vi "KGN Set Pump Concentrations.vi"(6 "Pump Concentrations-Cluster":T1(array[cluster]), 7 "scaling":dbl=1000000.0, 8 "Fehler (Eingang, kein Fehler)":errorcluster, 9 "Info Cluster":T2, 10 "VISA-Referenz (Eingang)":refnum<visa-resource-name>, 11 "device (Eingang)":u32) -> (0 "Fehler (Ausgang)":errorcluster, 1 "Info Cluster out":T2, 2 "VISA-Referenz (Ausgang)":refnum<visa-resource-name>, 3 "dup device (Ausgang)":u32, 4 "Kommandos gesendet":string)   [LabVIEW 2020, in "Linearisierung v2.lvlib" / "Gasteiler.lvlib" / "HovaCAL_Interface.lvlib" / "KGN.lvlib" / "KGN GUI Set.lvlib"]
uses:
  KGN GUI Set.lvlib
  Controls/Info Cluster.ctl
  set/set.lvlib
  Controls/Controls.lvlib
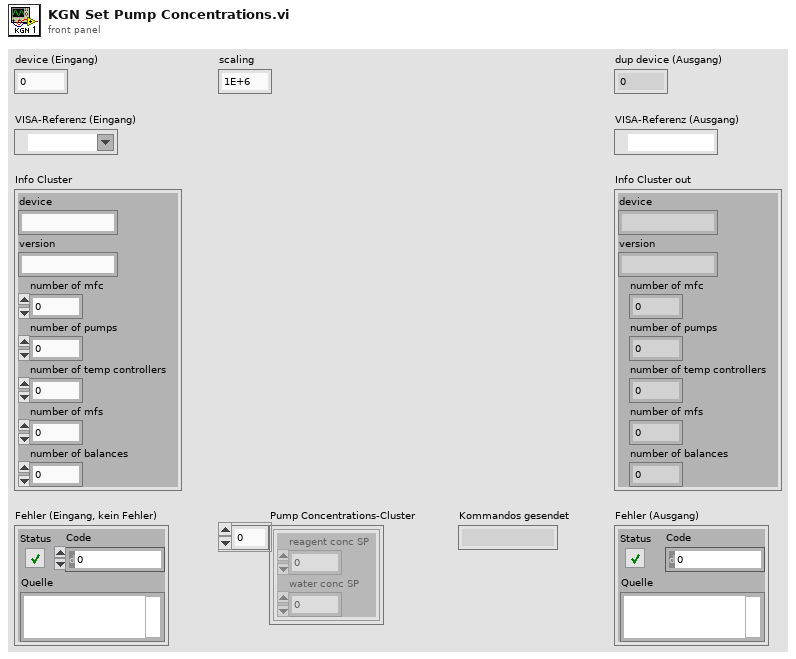
[diagram p1: front panel]
types:
  T1 = cluster{"reagent conc SP":dbl, "water conc SP":dbl}[]
  T2 = typedef "Linearisierung v2.lvlib/Gasteiler.lvlib/HovaCAL_Interface.lvlib/Controls.lvlib/Info Cluster.ctl" = cluster{"device":string, "version":string, "number of mfc":i32, "number of pumps":i32, "number of temp controllers":i32, "number of mfs":i32, "number of balances":i32}
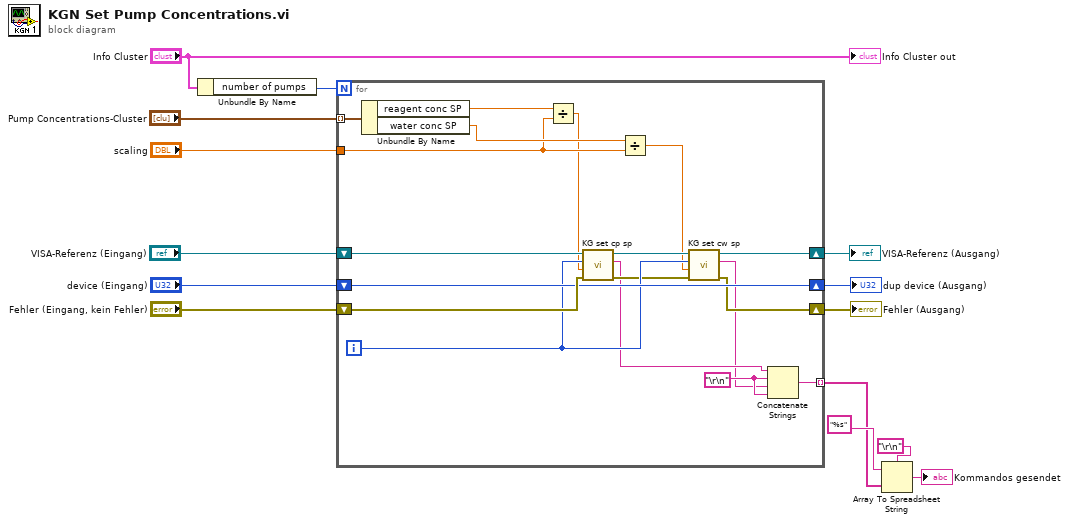
[diagram p0: block diagram]
diagram:
  n1 = Unbundle By Name("Info Cluster") -> ("number of pumps"=w9:i32)
  n2 = for {
    N: w9 -> [_]
    shift-right: [w31] -> w12
    shift-left: "device (Eingang)" -> [w31]
    shift-right: [w30] -> w11
    shift-left: "Fehler (Eingang, kein Fehler)" -> [w32]
    tunnel: "scaling" -> [w20]
    tunnel: "Pump Concentrations-Cluster" -> [w28] mode=indexing
    shift-right: [w25] -> w5
    shift-left: "VISA-Referenz (Eingang)" -> [w26]
    tunnel: [w15] -> w2 mode=indexing
    i -> [w29]
    w18 = "\r\n"
    n3 = Unbundle By Name(w28) -> ("reagent conc SP"=w21:dbl, "water conc SP"=w27:dbl)
    n4 = Divide(x=w21, y=w20) -> (x/y=w19:dbl)
    n5 = call "KG set cp sp.vi"("Fehler (Eingang, kein Fehler)"=w32, "Concentration"=w19, "pump"=w29, "VISA-Ressourcenname"=w26) -> ("Fehler (Ausgang)"=w23:errorcluster, "Kommando gesendet"=w17:string, "VISA-Ressourcenname (Ausgang)"=w24:refnum<visa-resource-name>)  [unwired: 5 in]
    n6 = Divide(x=w27, y=w20) -> (x/y=w22:dbl)
    n7 = call "KG set cw sp.vi"("Fehler (Eingang, kein Fehler)"=w23, "Concentration"=w22, "pump"=w29, "VISA-Ressourcenname"=w24) -> ("Fehler (Ausgang)"=w30:errorcluster, "Kommando gesendet"=w16:string, "VISA-Ressourcenname (Ausgang)"=w25:refnum<visa-resource-name>)  [unwired: 5 in]
    n8 = Concatenate Strings(w17, w18, w16, w18) -> (w15:string)
  }
  "dup device (Ausgang)" <- w12
  "Fehler (Ausgang)" <- w11
  "VISA-Referenz (Ausgang)" <- w5
  n9 = Array To Spreadsheet String(delimiter (Tab)="\r\n", array=w2, 3:"%s" ("Format-String")) -> (spreadsheet string=→"Kommandos gesendet":string)
  "Info Cluster out" <- "Info Cluster"
